vi "04Foot_Dev.vi"() -> ()   [LabVIEW 2020]
uses:
  <vilib>/DAQmx/read.llb/DAQmx Read (Digital 1D U8 1Chan NSamp).vi
  <vilib>/Instr/_visa.llb/VISA Configure Serial Port (Serial Instr).vi
  <vilib>/Utility/file.llb/Read Delimited Spreadsheet (I64).vi
  <vilib>/DAQmx/create/channels.llb/DAQmx Create Channel (DI-Digital Input).vi
  <vilib>/DAQmx/configure/timing.llb/DAQmx Timing (Change Detection).vi
  <vilib>/DAQmx/miscellaneous.llb/DAQmx Fill In Error Info.vi
panel:
  out "MPH READ 2":u8
  in  "Tab Control":enum32{"Page 1", "Page 2", "Page 3"}(tab)
  out "NEXT INC":u16 max=12 step=1
  out "INC":u16 max=12 step=1
  out "NEXT DURATION":u16
  out "NEXT MPH":u16 max=12 step=1
  out "Time Left":u16 format="%#.0f"
  out "ESTOP":bool
  in  "ESTOP RESUME":bool
  out "MPH":u16 max=12 step=1
  out "incline":u16[](array[numeric])
  out "ESTOP2":bool
  out "Report Location":path
  in  "TestScript":path=path "C:/LabView Computer Backup SEAL2788/DonP_TRM500/FootTimeInc.txt"
  out "Waveform Graph":dbl[](graph)
  out "speed":u16[](array[numeric])
  out "time":u16[](array[numeric])
  out "dwell":u16[](array[numeric])
  out "step":i32
  out "arraysize":i32
  out "x-y":u32
  out "appended path":path
  out "stopping":bool
  out "String":string
  in  "stop":bool
  out "MPH READ":u8
  in  "Serial Port":refnum<visa-resource-name>="COM8"
  in  "lines":tag="cDAQ1Mod1/port0/line0"
  out "Enum":T1(ring)
  out "FootPath":path
  out "Array":T2(array[cluster])
  out "size(s)":i32
  out "FootPathRef":refnum<file>
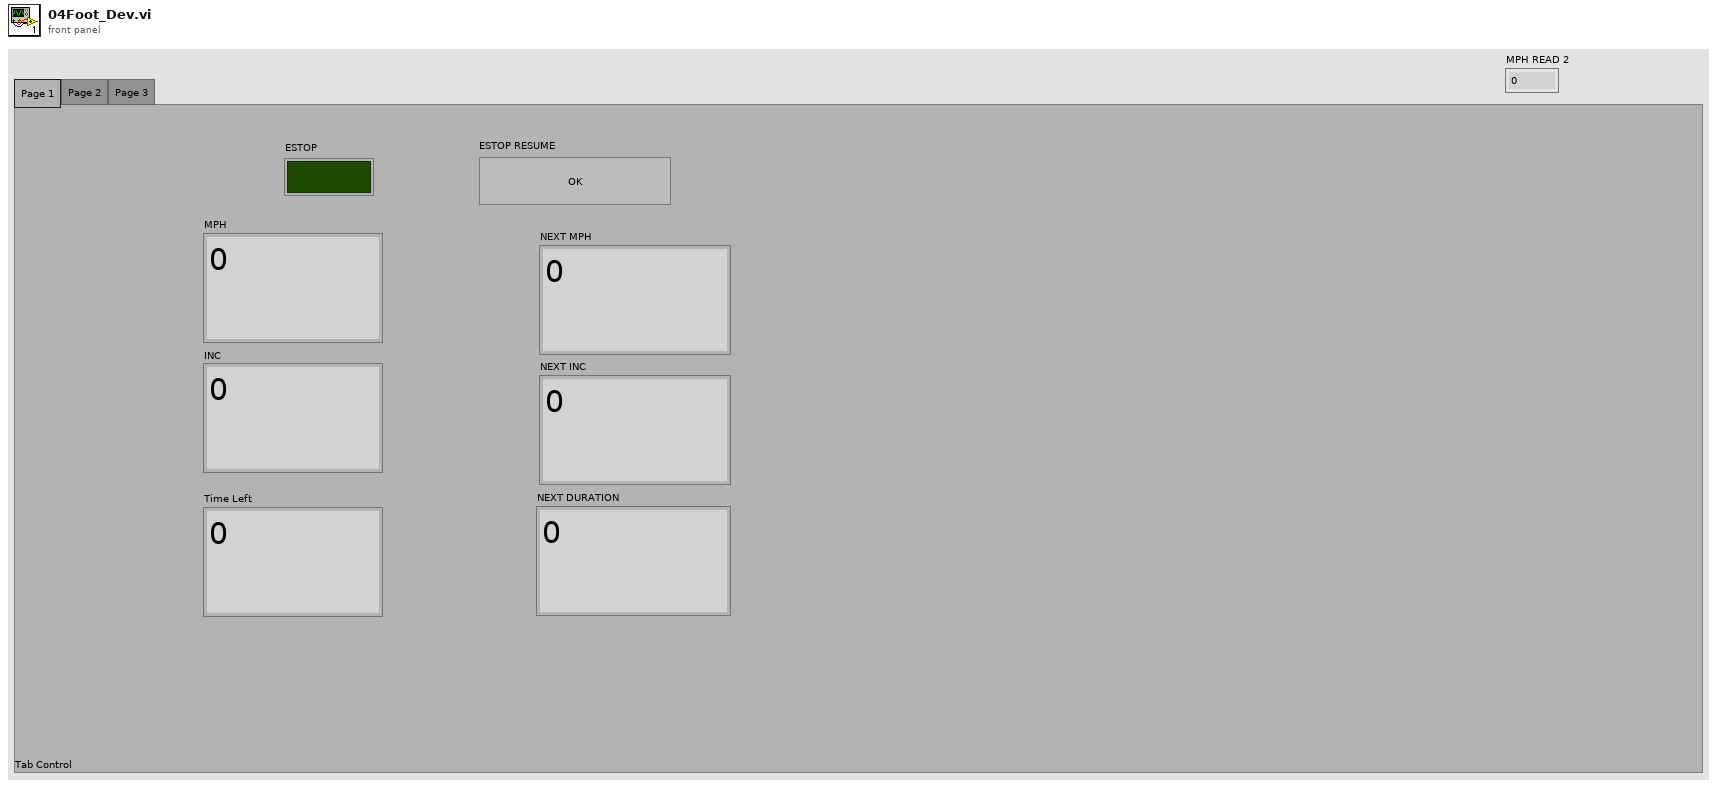
[diagram p1: front panel]
types:
  T1 = enum16{"Initialize", "SetMPH", "GetData", "CheckTiming", "CompressWave", "StartDAQ", "StopDAQ", "Dwell", "WaitforMPH", "ESTOP Wait", "ESTOP Resume"}
  T2 = cluster{"Trigger Time":timestamp, "MPH":dbl, "INC":dbl}[]
  T3 = cluster{"seconds since 1Jan1904":timestamp, "MPH":dbl, "INC":dbl}[]
  T4 = cluster{"Time":timestamp, "MPH":dbl, "INC":dbl}[]
  T5 = enum16{"Initialize", "SetMPH", "GetData", "CheckTiming", "CompressWave", "StartDAQ"}
  T6 = enum16{"Initialize", "SetMPH", "GetData", "CheckTiming", "CompressWave", "StartDAQ", "StopDAQ"}
  T7 = enum16{"Initialize", "SetMPH", "GetData", "CheckTiming", "CompressWave", "StartDAQ", "StopDAQ", "Dwell", "WaitforMPH"}
  T8 = cluster{"seconds since 1Jan1904":timestamp, "MPH":u16, "INC":u16}
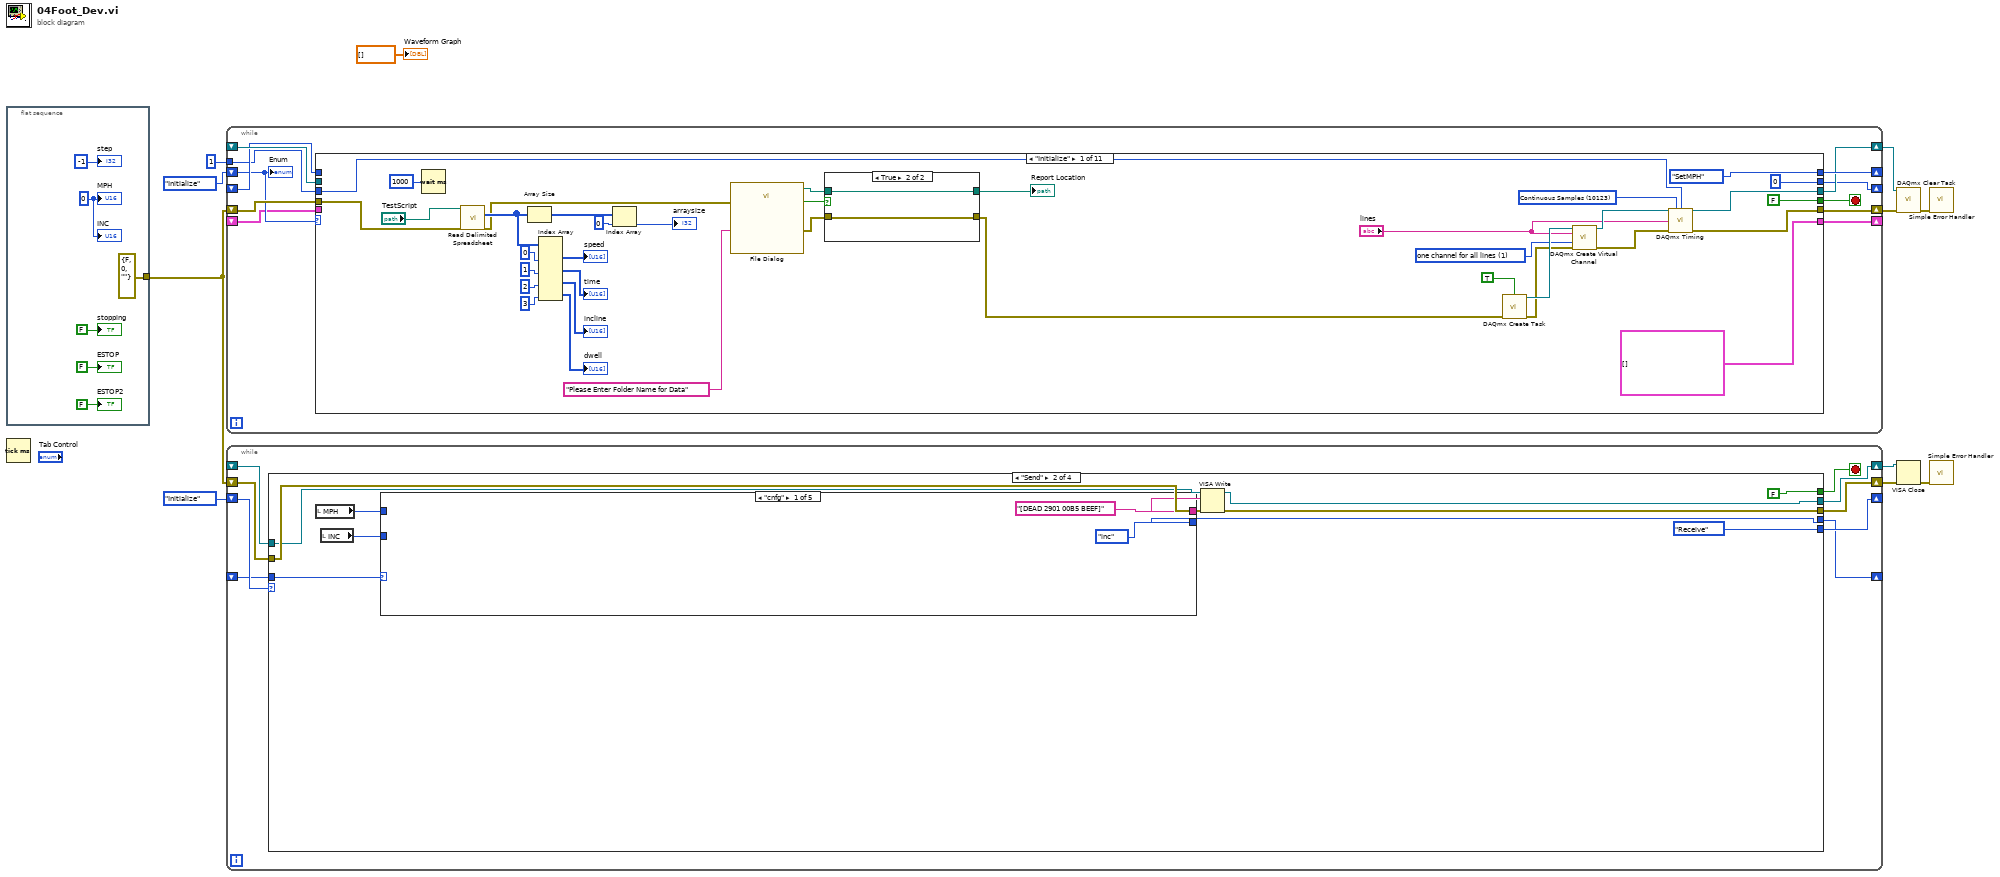
[diagram p0: block diagram]
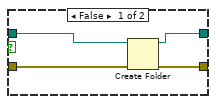
[diagram p2: hidden frame]
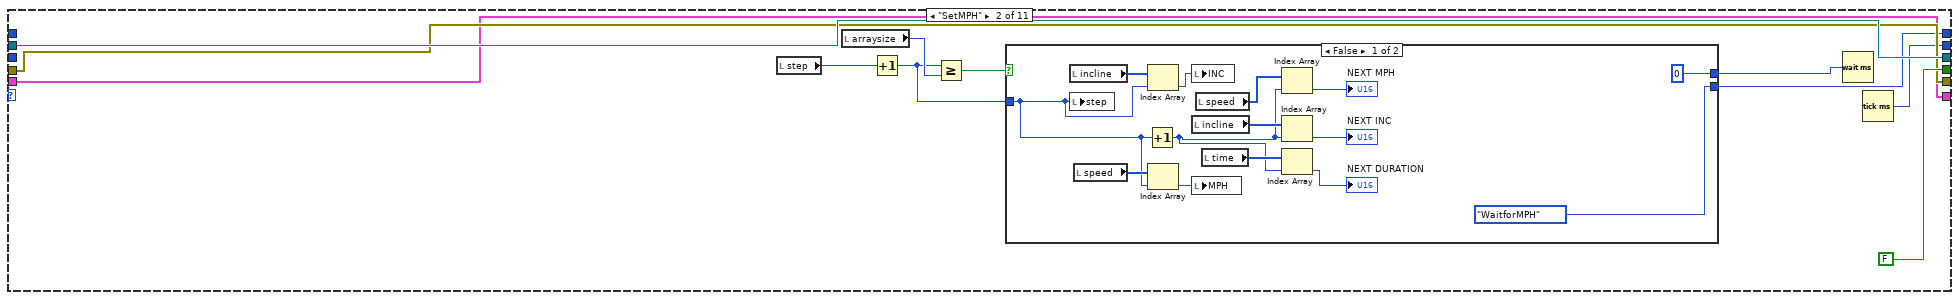
[diagram p3: hidden frame]
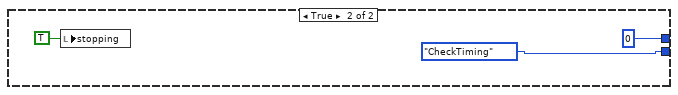
[diagram p4: hidden frame]
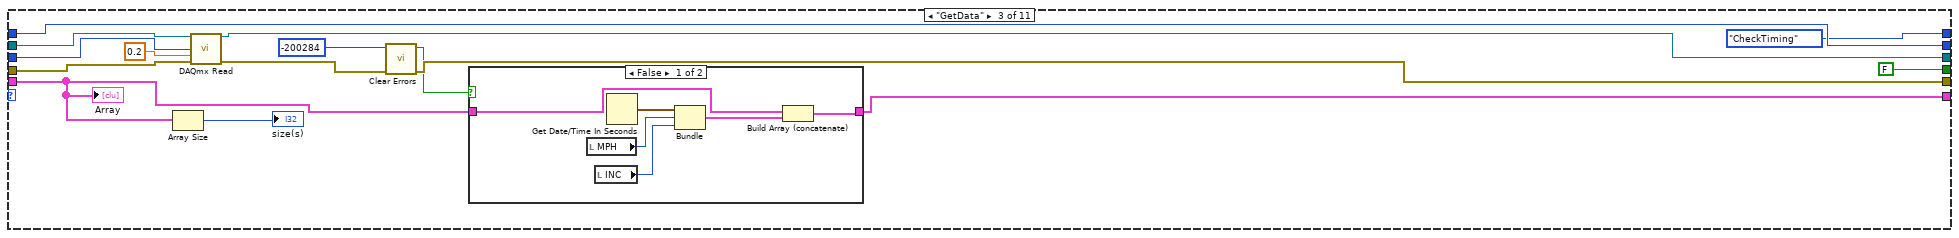
[diagram p5: hidden frame]
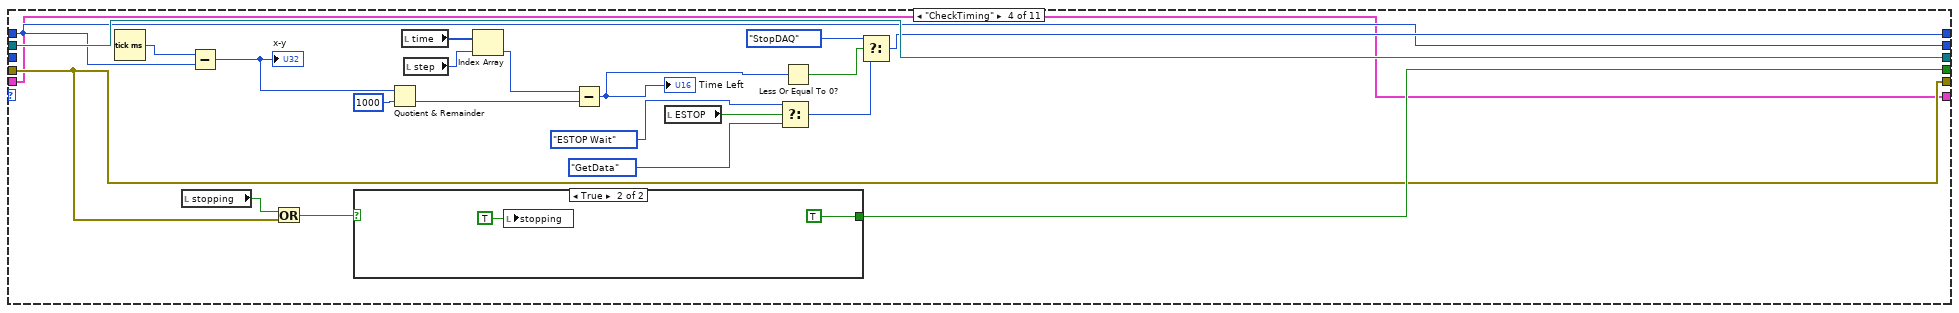
[diagram p7: hidden frame]
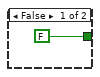
[diagram p8: hidden frame]
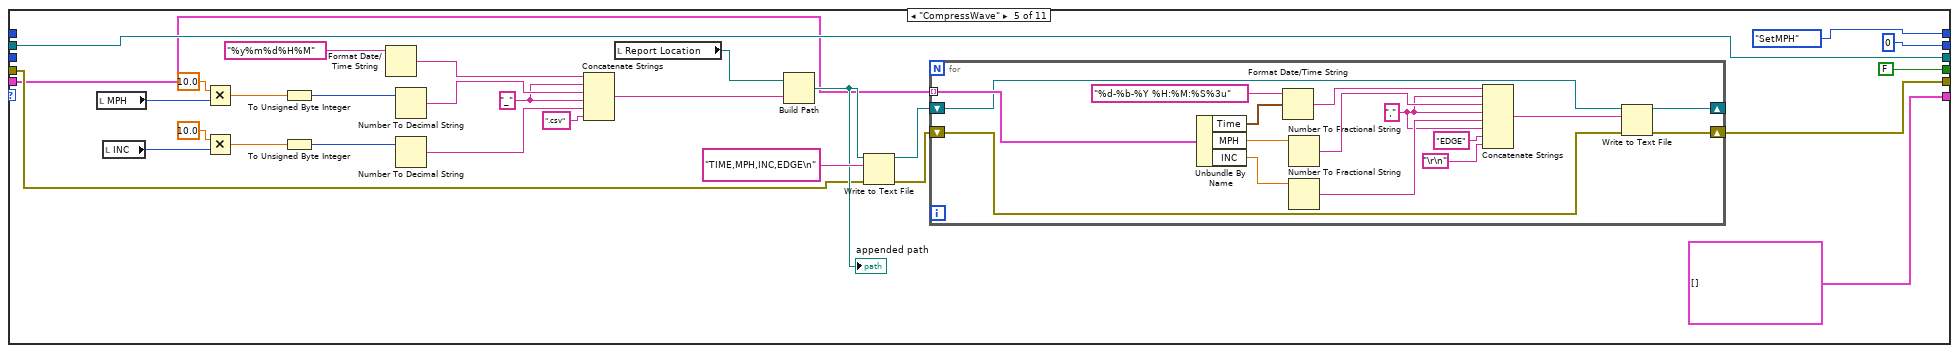
[diagram p9: hidden frame]
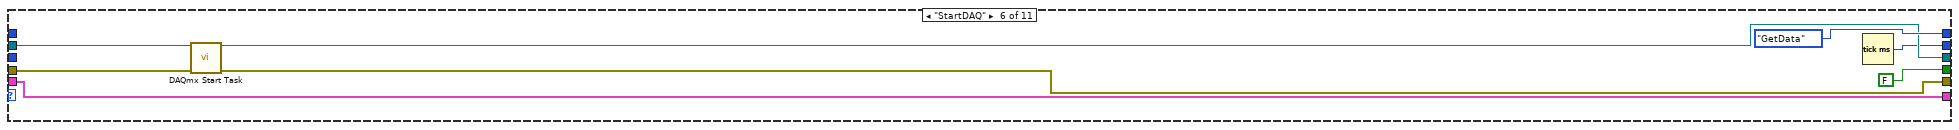
[diagram p10: hidden frame]
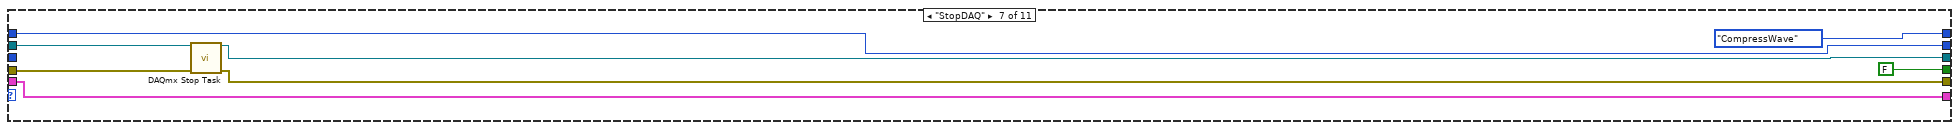
[diagram p11: hidden frame]
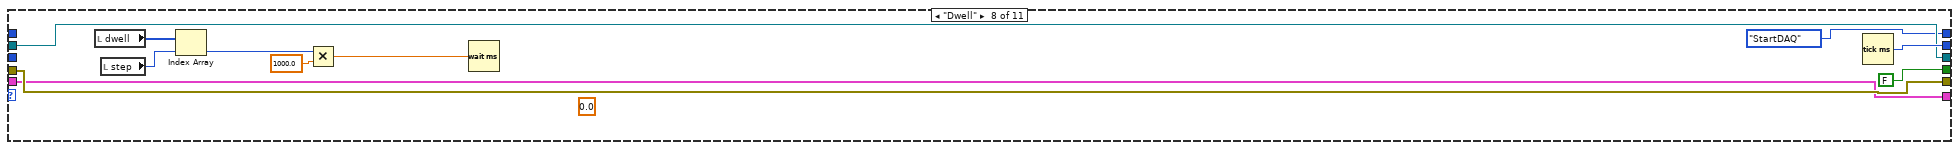
[diagram p12: hidden frame]
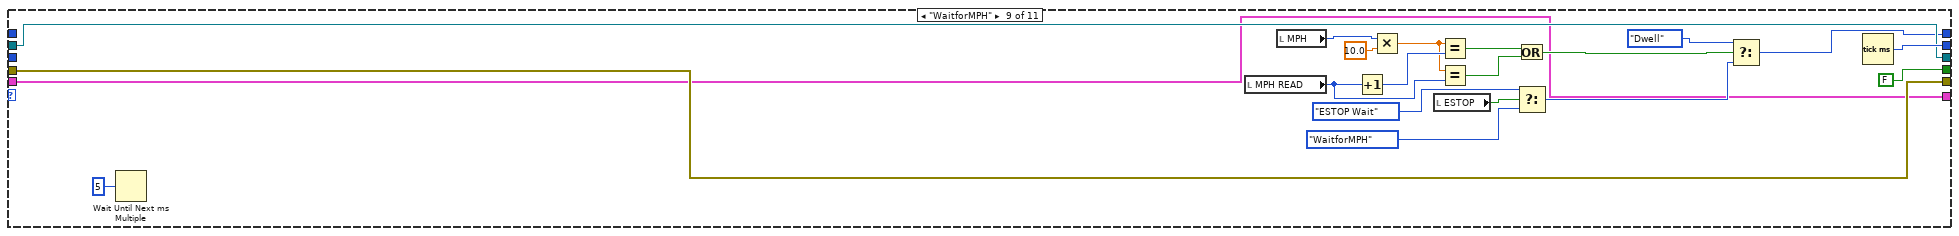
[diagram p13: hidden frame]
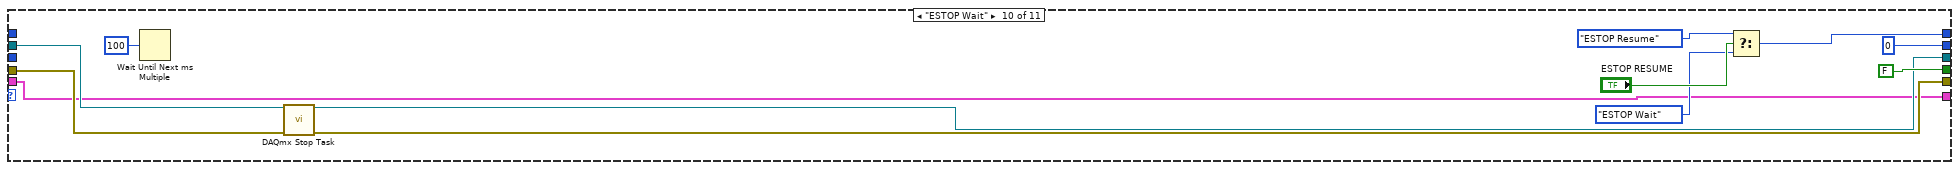
[diagram p14: hidden frame]
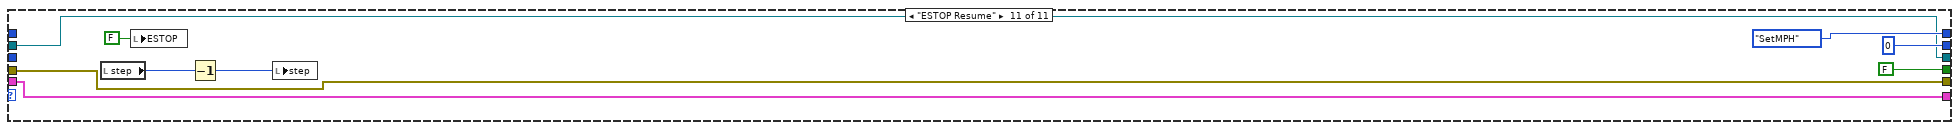
[diagram p15: hidden frame]
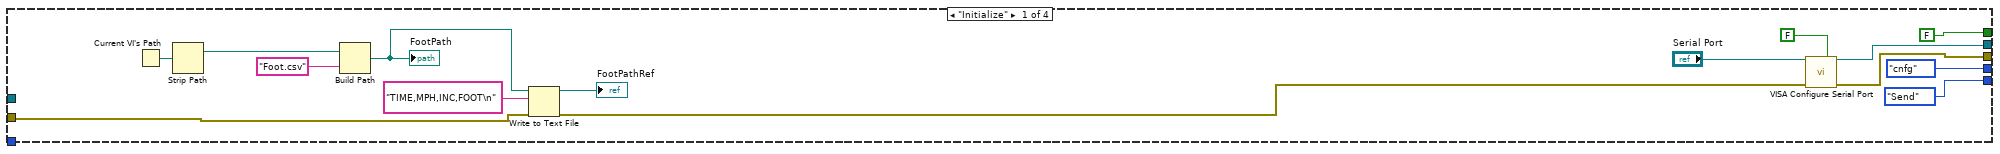
[diagram p16: hidden frame]
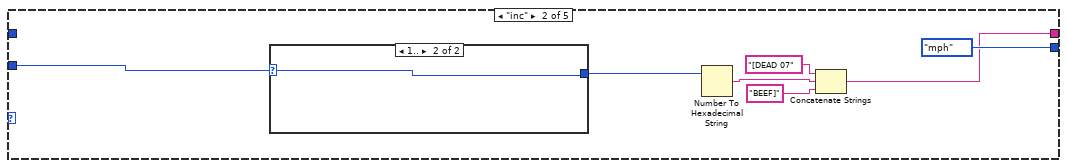
[diagram p17: hidden frame]
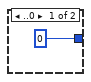
[diagram p18: hidden frame]
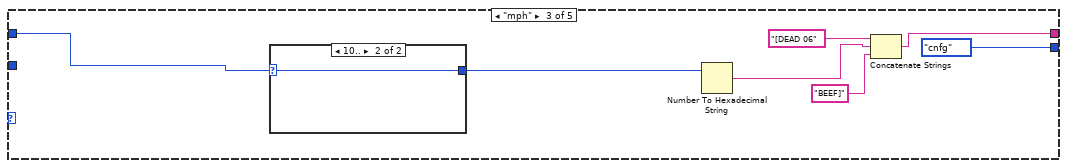
[diagram p19: hidden frame]
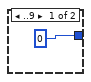
[diagram p20: hidden frame]
diagram:
  n1 = flat-sequence {
    tunnel: [errorcluster {"status"=FALSE, "code"=0, "source"=""} ("error constant")] -> w3
    frame #0 {
      w12 = u16 0 ("MPH")
      "stopping" <- FALSE ("stopping")
      "MPH" <- w12
      "step" <- -1 ("step")
      "ESTOP" <- FALSE ("ESTOP")
      "ESTOP2" <- FALSE ("ESTOP2")
      "INC" <- w12
    }
  }
  n2 = Tick Count (ms)() -> ()  [unwired: 1 out]
  n3 = while {
    shift-right: [w29] -> _
    shift-left: T1."Initialize" -> [w20]
    shift-right: [w27] -> w5
    shift-left: _ -> [w25]
    shift-right: [w26] -> w6
    shift-left: w3 -> [w24]
    shift-right: [w23] -> _
    shift-left: _ -> [w22]
    tunnel: 1 ("samples per channel") -> [w21]
    shift-right: [w18] -> _
    shift-left: _ -> [w19]
    stop <- w28 stop-if-true
    n4 = case shown="\"Initialize\"" w20 {
      tunnel: [T1."SetMPH" w79 T1."CheckTiming" ("f") w139 T1."SetMPH" T5."GetData" T6."CompressWave" T7."StartDAQ" w231 w245 T1."SetMPH" ("f")] -> w29
      tunnel: [FALSE FALSE FALSE w143 FALSE FALSE FALSE FALSE FALSE FALSE FALSE] -> w28
      tunnel: [w35 w81 w107 w144 w166 w196 w204 w217 w237 w241 w254] -> w27
      tunnel: [w36 w80 w106 w140 w148 w197 w203 w216 w236 w240 w255] -> w26
      tunnel: w25 -> [_ w81 w110 w144 w166 w195 w206 w217 w237 w243 w254]
      tunnel: w24 -> [w60 w80 w109 w140 w152 w194 w205 w216 w236 w242 w255]
      tunnel: [u32 0 w73 w114 w127 u32 0 w192 w201 w218 w238 u32 0 ("millisecond timer value") u32 0 ("millisecond timer value")] -> w23
      tunnel: w22 -> [_ _ w114 w127 _ _ w201 _ _ _ _]
      tunnel: w21 -> [w57 _ w108 _ _ _ _ _ _ _ _]
      tunnel: w19 -> [_ w74 w102 w126 w151 w193 w200 w208 w219 w239 w251]
      tunnel: [T3 [] w74 w105 w126 T4 [] w193 w200 w208 w219 w239 w251] -> w18
      frame "Initialize" {
        w56 = 10123 items=["Finite Samples"=10178, "Continuous Samples"=10123, "Hardware Timed Single Point"=12522] ("sample mode")
        w64 = 1 items=["one channel for each line", "one channel for all lines"] ("line grouping")
        n5 = Wait (ms)(milliseconds to wait=u32 1000) -> ()  [unwired: 1 out]
        n6 = call-poly <vilib>:"Read Delimited Spreadsheet.vi"("file path (dialog if empty)"="TestScript", "error in (no error)"=w60) -> ("all rows"=w47:i64[][], "error out"=w45:errorcluster)  [unwired: 8 in, 4 out]
        n7 = Array Size(array=w47) -> (size(s)=w50:i32[])
        n8 = Index Array(array=w47, index (col) #1=0 ("disabled index (col)"), index (col) #2=1 ("index (col)"), index (col) #3=2 ("index (col)"), index (col) #4=3 ("index (col)")) -> (element #1=→"speed":i64[], element #2=→"time":i64[], element #3=→"incline":i64[], element #4=→"dwell":i64[])  [unwired: 4 in]
        n9 = Index Array(array=w50, index=0) -> (element=→"arraysize":i32)
        n10 = call "File Dialog"("prompt"="Please Enter Folder Name for Data", "error in"=w45) -> ("selected path"=w41:path, "exists"=w43:bool, "error out"=w42:errorcluster)  [unwired: 10 in, 1 out]
        n11 = case shown="True" w43 {
          tunnel: w42 -> [w70 w71]
          tunnel: w41 -> [w69 w72]
          tunnel: [w68 w71] -> w40
          tunnel: [w67 w72] -> w39
          frame False {
            n12 = Create Folder(path (use dialog)=w69, error in=w70) -> (created path=w67:path, error out=w68:errorcluster)  [unwired: 1 in, 1 out]
          }
          frame True {
          }
        }
        "Report Location" <- w39
        n13 = call <vilib>:"DAQmx Create Task.vi"("auto cleanup"=TRUE, "error in"=w40) -> ("task out"=w66:refnum<k21>, "error out"=w65:errorcluster)  [unwired: 12 in]
        n14 = call-poly <vilib>:"DAQmx Create Virtual Channel.vi"("task in"=w66, "lines"="lines", "line grouping"=w64, "error in"=w65) -> ("task out"=w58:refnum<k21>, "error out"=w59:errorcluster)  [unwired: 10 in]
        n15 = call-poly <vilib>:"DAQmx Timing.vi"("task/channels in"=w58, "sample mode"=w56, "samples per channel"=w57, "rising edge physical channels"="lines", "error in"=w59) -> ("task out"=w35:refnum<k21>, "error out"=w36:errorcluster)  [unwired: 9 in]
      }
      frame "SetMPH" {
        n16 = local read "step"() -> (w76:i32)
        n17 = local read "arraysize"() -> (w78:i32)
        n18 = Increment(x=w76) -> (x+1=w75:i32)
        n19 = Greater Or Equal?(x=w75, y=w78) -> (x >= y?=w77:bool)
        n20 = case shown="False" w77 {
          tunnel: [u32 0 ("milliseconds to wait") u32 0 ("milliseconds to wait")] -> w82
          tunnel: [T1."WaitforMPH" T1."CheckTiming"] -> w79
          tunnel: w75 -> [w86 _]
          frame False {
            n21 = local read "incline"() -> (w87:u16[])
            n22 = local write "step"(w86) -> ()
            n23 = local read "speed"() -> (w96:u16[])
            n24 = Increment(x=w86) -> (x+1=w88:i32)
            n25 = Index Array(array=w87, index=w86) -> (element=w85:u16)
            n26 = Index Array(array=w96, index=w86) -> (element=w95:u16)
            n27 = local write "INC"(w85) -> ()
            n28 = local read "incline"() -> (w89:u16[])
            n29 = local write "MPH"(w95) -> ()
            n30 = local read "speed"() -> (w94:u16[])
            n31 = local read "time"() -> (w91:u16[])
            n32 = Index Array(array=w94, index=w88) -> (element=→"NEXT MPH":u16)
            n33 = Index Array(array=w89, index=w88) -> (element=→"NEXT INC":u16)
            n34 = Index Array(array=w91, index=w88) -> (element=→"NEXT DURATION":u16)
          }
          frame True {
            n35 = local write "stopping"(TRUE ("stopping")) -> ()
          }
        }
        n36 = Wait (ms)(milliseconds to wait=w82) -> ()  [unwired: 1 out]
        n37 = Tick Count (ms)() -> (millisecond timer value=w73:u32)
      }
      frame "GetData" {
        n38 = Array Size(array=w102) -> (size(s)=→"size(s)":i32)
        n39 = call-poly <vilib>:"DAQmx Read.vi"("task/channels in"=w110, "number of samples per channel"=w108, "timeout"=0.2, "error in"=w109) -> ("task out"=w107:refnum<k21>, "error out"=w111:errorcluster)  [unwired: 9 in, 1 out]
        n40 = call <vilib>:"Clear Errors.vi"("error in (no error)"=w111, "specific error code to clear (0: all)"=-200284) -> ("error out"=w106:errorcluster, "specific error cleared?"=w103:bool)  [unwired: 4 in]
        n41 = case shown="False" w103 {
          tunnel: [w121 w122] -> w105
          tunnel: w102 -> [w120 w122]
          frame False {
            n42 = local read "MPH"() -> (w117:u16)
            n43 = local read "INC"() -> (w116:u16)
            n44 = Get Date/Time In Seconds() -> (seconds since 1Jan1904=w119:timestamp)
            n45 = Bundle("seconds since 1Jan1904"=w119, "MPH"=w117, "INC"=w116) -> (w118:T8)  [unwired: 1 in]
            n46 = Build Array (concatenate)(w120, w118) -> (w121:T3)
          }
          frame True {
          }
        }
        "Array" <- w102
      }
      frame "CheckTiming" {
        n47 = Tick Count (ms)() -> (millisecond timer value=w128:u32)
        n48 = local read "stopping"() -> (w142:bool)
        n49 = Subtract(x=w128, y=w127) -> (x-y=w125:u32)
        "x-y" <- w125
        n50 = Or(x=w142, y=w140) -> (x .or. y?=w141:bool)
        n51 = case shown="True" w141 {
          tunnel: [FALSE TRUE] -> w143
          frame False {
          }
          frame True {
            n52 = local write "stopping"(TRUE ("stopping")) -> ()
          }
        }
        n53 = Quotient & Remainder(x=w125, y=u32 1000) -> (floor(x/y)=w123:u32)  [unwired: 1 out]
        n54 = local read "time"() -> (w138:u16[])
        n55 = local read "step"() -> (w137:i32)
        n56 = Index Array(array=w138, index=w137) -> (element=w131:u16)
        n57 = Subtract(x=w131, y=w123) -> (x-y=w130:u32)
        "Time Left" <- w130
        n58 = local read "ESTOP"() -> (w134:bool)
        n59 = Select(t=T1."ESTOP Wait", s=w134, f=T1."GetData") -> (s? t:f=w132:T1)
        n60 = Less Or Equal To 0?(x=w130) -> (x <= 0?=w129:bool)
        n61 = Select(t=T1."StopDAQ", s=w129, f=w132) -> (s? t:f=w139:T1)
      }
      frame "CompressWave" {
        w160 = "_" ("string")
        n62 = local read "MPH"() -> (w167:u16)
        n63 = local read "INC"() -> (w156:u16)
        n64 = Multiply(x=10.0, y=w167) -> (x*y=w170:dbl)
        n65 = Multiply(x=10.0, y=w156) -> (x*y=w158:dbl)
        n66 = To Unsigned Byte Integer(number=w170) -> (unsigned 8bit integer=w169:u8)
        n67 = To Unsigned Byte Integer(number=w158) -> (unsigned 8bit integer=w157:u8)
        n68 = Format Date/Time String(time format string (%c)="%y%m%d%H%M") -> (date/time string=w163:string)  [unwired: 2 in]
        n69 = Number To Decimal String(number=w169) -> (decimal integer string=w168:string)  [unwired: 1 in]
        n70 = Number To Decimal String(number=w157) -> (decimal integer string=w155:string)  [unwired: 1 in]
        n71 = Concatenate Strings(w163, w160, w168, w160, w155, ".csv" ("string")) -> (w172:string)
        n72 = local read "Report Location"() -> (w165:path)
        n73 = Build Path(base path=w165, name or relative path=w172) -> (appended path=w153:path)
        "appended path" <- w153
        n74 = Write to Text File(file (use dialog)=w153, text="TIME,MPH,INC,EDGE\n", error in=w152) -> (refnum out=w150:refnum<file>, error out=w149:errorcluster)  [unwired: 1 in, 1 out]
        n75 = for {
          tunnel: w151 -> [w191] mode=indexing
          shift-right: [w177] -> _
          shift-left: w150 -> [w180]
          shift-right: [w176] -> w148
          shift-left: w149 -> [w179]
          w185 = ","
          n76 = Unbundle By Name(w191) -> ("Time"=w183:timestamp, "MPH"=w182:dbl, "INC"=w181:dbl)
          n77 = Format Date/Time String(time format string (%c)="%d-%b-%Y %H:%M:%S%3u", seconds (now)=w183) -> (date/time string=w189:string)  [unwired: 1 in]
          n78 = Number To Fractional String(number=w182) -> (F-format string=w188:string)  [unwired: 3 in]
          n79 = Number To Fractional String(number=w181) -> (F-format string=w187:string)  [unwired: 3 in]
          n80 = Concatenate Strings(w189, w185, w188, w185, w187, w185, "EDGE", "\r\n") -> (w178:string)
          n81 = Write to Text File(file (use dialog)=w180, text=w178, error in=w179) -> (refnum out=w177:refnum<file>, error out=w176:errorcluster)  [unwired: 1 in, 1 out]
        }
      }
      frame "StartDAQ" {
        n82 = call <vilib>:"DAQmx Start Task.vi"("task/channels in"=w195, "error in"=w194) -> ("task out"=w196:refnum<k21>, "error out"=w197:errorcluster)  [unwired: 12 in]
        n83 = Tick Count (ms)() -> (millisecond timer value=w192:u32)
      }
      frame "StopDAQ" {
        n84 = call <vilib>:"DAQmx Stop Task.vi"("task/channels in"=w206, "error in"=w205) -> ("task out"=w204:refnum<k21>, "error out"=w203:errorcluster)  [unwired: 12 in]
      }
      frame "Dwell" {
        (unwired) 0.0
        n85 = local read "dwell"() -> (w214:u16[])
        n86 = local read "step"() -> (w213:i32)
        n87 = Index Array(array=w214, index=w213) -> (element=w212:u16)
        n88 = Multiply(x=w212, y=1000.0) -> (x*y=w210:dbl)
        n89 = Wait (ms)(milliseconds to wait=w210) -> ()  [unwired: 1 out]
        n90 = Tick Count (ms)() -> (millisecond timer value=w218:u32)
      }
      frame "WaitforMPH" {
        n91 = Wait Until Next ms Multiple(millisecond multiple=u32 5) -> ()  [unwired: 1 out]
        n92 = local read "MPH READ"() -> (w223:u8)
        n93 = local read "MPH"() -> (w234:u16)
        n94 = Increment(x=w223) -> (x+1=w232:u8)
        n95 = Multiply(x=w234, y=10.0) -> (x*y=w224:dbl)
        n96 = local read "ESTOP"() -> (w229:bool)
        n97 = Equal?(x=w224, y=w232) -> (x = y?=w221:bool)
        n98 = Equal?(x=w224, y=w223) -> (x = y?=w222:bool)
        n99 = Or(x=w221, y=w222) -> (x .or. y?=w220:bool)
        n100 = Select(t=T1."ESTOP Wait", s=w229, f=T1."WaitforMPH") -> (s? t:f=w226:T1)
        n101 = Select(t=T1."Dwell", s=w220, f=w226) -> (s? t:f=w231:T1)
        n102 = Tick Count (ms)() -> (millisecond timer value=w238:u32)
      }
      frame "ESTOP Wait" {
        n103 = Wait Until Next ms Multiple(millisecond multiple=u32 100) -> ()  [unwired: 1 out]
        n104 = call <vilib>:"DAQmx Stop Task.vi"("task/channels in"=w243, "error in"=w242) -> ("task out"=w241:refnum<k21>, "error out"=w240:errorcluster)  [unwired: 12 in]
        n105 = Select(t=T1."ESTOP Resume", s="ESTOP RESUME", f=T1."ESTOP Wait") -> (s? t:f=w245:T1)
      }
      frame "ESTOP Resume" {
        n106 = local read "step"() -> (w259:i32)
        n107 = local write "ESTOP"(FALSE ("ESTOP")) -> ()
        n108 = Decrement(x=w259) -> (x-1=w258:i32)
        n109 = local write "step"(w258) -> ()
      }
    }
    "Enum" <- w20
  }
  n110 = while {
    shift-right: [w264] -> w9
    shift-left: w3 -> [w268]
    shift-right: [w265] -> w10
    shift-left: _ -> [w267]
    shift-right: [w263] -> _
    shift-left: enum16{"Initialize", "Send", "Receive", "Error"}."Initialize" -> [w266]
    shift-right: [w262] -> _
    shift-left: _ -> [w261]
    stop <- w260 stop-if-true
    n111 = case shown="\"Send\"" w266 {
      tunnel: w268 -> [w271 w292 w339 w380]
      tunnel: w267 -> [_ w291 w338 w384]
      tunnel: [w281 w294 w337 w384] -> w265
      tunnel: [w280 w293 w319 w380] -> w264
      tunnel: [enum16{"Initialize", "Send", "Receive", "Error"}."Send" enum16{"Initialize", "Send", "Receive", "Error"}."Receive" enum16{"Initialize", "Send", "Receive", "Error"}."Error" enum16{"Initialize", "Send", "Receive", "Error"}."Send"] -> w263
      tunnel: [enum16{"cnfg", "inc", "mph", "err", "RSET"}."cnfg" w288 w327 w385] -> w262
      tunnel: w261 -> [_ w289 w332 w385]
      tunnel: [FALSE FALSE FALSE w379] -> w260
      frame "Initialize" {
        n112 = Current VI's Path() -> (path=w276:path)
        n113 = Strip Path(path=w276) -> (stripped path=w275:path)  [unwired: 1 out]
        n114 = Build Path(base path=w275, name or relative path="Foot.csv") -> (appended path=w272:path)
        "FootPath" <- w272
        n115 = Write to Text File(file (use dialog)=w272, text="TIME,MPH,INC,FOOT\n", error in=w271) -> (refnum out=→"FootPathRef":refnum<file>, error out=w270:errorcluster)  [unwired: 1 in, 1 out]
        n116 = call-poly "VISA Configure Serial Port"("VISA resource name"="Serial Port", "Enable Termination\nChar (T)"=FALSE ("Enable Termination\nChar (T)"), "error in (no error)"=w270) -> ("VISA resource name out"=w281:refnum<visa-resource-name>, "error out"=w280:errorcluster)  [unwired: 11 in]
      }
      frame "Send" {
        n117 = local read "MPH"() -> (w285:u16)
        n118 = local read "INC"() -> (w284:u16)
        n119 = case shown="\"cnfg\"" w289 {
          tunnel: ["[DEAD 2901 00B5 BEEF]" w298 w307 "[err]" "[RSET]"] -> w290
          tunnel: w285 -> [_ _ w306 _ _]
          tunnel: [enum16{"cnfg", "inc", "mph", "err", "RSET"}."inc" enum16{"cnfg", "inc", "mph", "err", "RSET"}."mph" enum16{"cnfg", "inc", "mph", "err", "RSET"}."cnfg" enum16{"cnfg", "inc", "mph", "err", "RSET"}."cnfg" enum16{"cnfg", "inc", "mph", "err", "RSET"}."cnfg"] -> w288
          tunnel: w284 -> [_ w297 _ _ _]
          frame "cnfg" {
          }
          frame "inc" {
            n120 = case shown="1.." w297 {
              selector: w297 -> [_ w305]
              tunnel: [u8 0 w305] -> w299
              frame ..0 {
              }
              frame 1.. {
              }
            }
            n121 = Number To Hexadecimal String(2:w299) -> (0:w302:string)  [unwired: 1 in]
            n122 = Concatenate Strings("[DEAD 07" ("string"), w302, "BEEF]" ("string")) -> (w298:string)
          }
          frame "mph" {
            n123 = case shown="10.." w306 {
              selector: w306 -> [_ w314]
              tunnel: [u8 0 w314] -> w308
              frame ..9 {
              }
              frame 10.. {
              }
            }
            n124 = Number To Hexadecimal String(2:w308) -> (0:w311:string)  [unwired: 1 in]
            n125 = Concatenate Strings("[DEAD 06" ("string"), w311, "BEEF]" ("string")) -> (w307:string)
          }
          frame "err" {
          }
          frame "RSET" {
          }
        }
        n126 = VISA Write(VISA resource name=w291, write buffer=w290, error in (no error)=w292) -> (VISA resource name out=w294:refnum<visa-resource-name>, error out=w293:errorcluster)  [unwired: 1 out]
      }
      frame "Receive" {
        n127 = flat-sequence {
          tunnel: w338 -> [w377]
          tunnel: [w377] -> w343
          frame #0 {
            n128 = Wait Until Next ms Multiple(millisecond multiple=u32 250) -> ()  [unwired: 1 out]
          }
        }
        n129 = property class="Serial Instr"(reference=w343, error in=w339) -> (reference out=w341:refnum<visa-resource-name>, error out=w342:errorcluster, "Bytes at Port"=w340:u32)
        n130 = VISA Read(VISA resource name=w341, byte count=w340, error in (no error)=w342) -> (VISA resource name out=w337:refnum<visa-resource-name>, read buffer=w323:string, error out=w344:errorcluster)  [unwired: 1 out]
        n131 = Match Pattern(string=w323, regular expression="\\[ESTOP:BAD\\]") -> (offset past match=w326:i32)  [unwired: 1 in, 3 out]
        n132 = Match Pattern(string=w323, regular expression="\\[err:") -> (offset past match=w333:i32)  [unwired: 1 in, 3 out]
        n133 = Match Pattern(string=w323, regular expression="\\[mph:") -> (after substring=w329:string, offset past match=w330:i32)  [unwired: 1 in, 2 out]
        n134 = Match Pattern(string=w323, regular expression="\\[foot:") -> (match substring=w321:string, after substring=w320:string, offset past match=w322:i32)  [unwired: 1 in, 1 out]
        n135 = case shown="Default" w330 {
          tunnel: w329 -> [w371 _]
          frame Default {
            n136 = Hexadecimal String To Number(string=w371, default (0uL)=u8 0 ("default (0 I32)")) -> (number=→"MPH READ" →"MPH READ 2":u8)  [unwired: 1 in, 1 out]
          }
          frame -1 {
          }
        }
        n137 = case shown="Default" w322 {
          tunnel: w321 -> [w361 _]
          tunnel: w320 -> [w363 _]
          tunnel: w344 -> [w351 w364]
          tunnel: [w348 w364] -> w319
          frame Default {
            w353 = ","
            n138 = Match Pattern(string=w363, regular expression="\\]") -> (before substring=w360:string, match substring=w359:string)  [unwired: 1 in, 2 out]
            n139 = Concatenate Strings(w361, w360, w359) -> (w352:string)
            n140 = local read "MPH"() -> (w347:u16)
            n141 = local read "INC"() -> (w346:u16)
            n142 = Format Date/Time String(time format string (%c)="%d-%b-%Y %H:%M:%S%3u") -> (date/time string=w357:string)  [unwired: 2 in]
            n143 = Number To Fractional String(number=w347) -> (F-format string=w356:string)  [unwired: 3 in]
            n144 = Number To Fractional String(number=w346) -> (F-format string=w355:string)  [unwired: 3 in]
            n145 = Concatenate Strings(w357, w353, w356, w353, w355, w353, w352, "\r\n") -> (w349:string)
            n146 = local read "FootPathRef"() -> (w350:refnum<file>)
            n147 = Write to Text File(file (use dialog)=w350, text=w349, error in=w351) -> (refnum out=w345:refnum<file>, error out=w348:errorcluster)  [unwired: 1 in, 1 out]
            n148 = local write "FootPathRef"(w345) -> ()
          }
          frame -1 {
          }
        }
        n149 = case shown="Default" w333 {
          tunnel: [enum16{"cnfg", "inc", "mph", "err", "RSET"}."RSET" w376] -> w328
          tunnel: w332 -> [_ w376]
          tunnel: w323 -> [w372 _]
          frame Default {
            (unwired) "%y%m%d%H%M" ("time format string (%c)")
            n150 = Format Date/Time String() -> (date/time string=w373:string)  [unwired: 3 in]
            n151 = Concatenate Strings(w373, w372) -> (→"String":string)
          }
          frame -1 {
          }
        }
        n152 = case shown="Default" w326 {
          tunnel: w328 -> [_ w368]
          tunnel: [enum16{"cnfg", "inc", "mph", "err", "RSET"}."RSET" w368] -> w327
          frame Default {
            n153 = local write "MPH"(0.0 ("MPH")) -> ()
            n154 = local write "ESTOP"(TRUE ("ESTOP")) -> ()
          }
          frame -1 {
          }
        }
      }
      frame "Error" {
        n155 = local read "stopping"() -> (w381:bool)
        n156 = Compound Arithmetic op=OR("stop", w381, w380) -> (w383:bool)
        n157 = case shown="True" w383 {
          tunnel: [FALSE TRUE] -> w379
          frame False {
          }
          frame True {
            n158 = local write "stopping"(TRUE ("stopping")) -> ()
          }
        }
      }
    }
  }
  n159 = call <vilib>:"DAQmx Clear Task.vi"("task in"=w5, "error in"=w6) -> ("error out"=w4:errorcluster)  [unwired: 13 in]
  n160 = VISA Close(VISA resource name=w10, error in (no error)=w9) -> (error out=w8:errorcluster)
  n161 = call <vilib>:"Simple Error Handler.vi"("error in (no error)"=w4) -> ()  [unwired: 4 in, 5 out]
  n162 = call <vilib>:"Simple Error Handler.vi"("error in (no error)"=w8) -> ()  [unwired: 4 in, 5 out]
  "Waveform Graph" <- dbl[] []
